vi "Factor multiply Parameter.vi"(9 "Factor to multiply":dbl[](array[numeric]), 10 "Z":i32[](array[numeric]), 11 "Param In":T1) -> (3 "Param Out":T1)   [LabVIEW 2023]
uses:
  control/Parameters.ctl
  c738a0e9-d9eb-444f-adff-f9f269ff3581.vi
  <vilib>/Comparison/Equal/Equal Functor/Equal Functor.lvclass
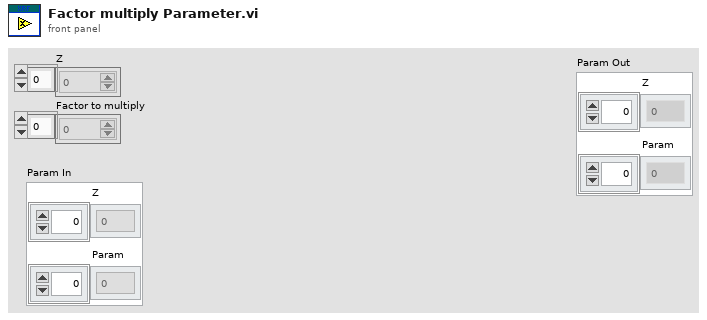
[diagram p1: front panel]
types:
  T1 = typedef "Parameters.ctl" = cluster{"Z":i32[], "Param":dbl[]}
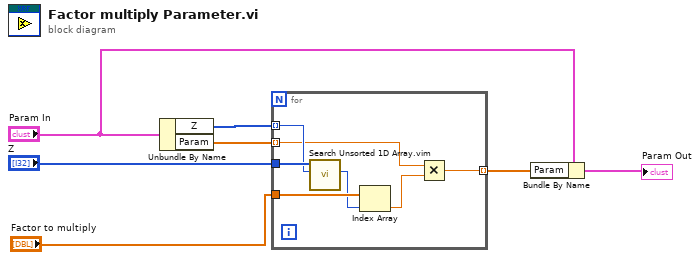
[diagram p0: block diagram]
diagram:
  n1 = Unbundle By Name("Param In") -> ("Z"=w5:i32[], "Param"=w4:dbl[])
  n2 = for {
    tunnel: "Z" -> [w13]
    tunnel: w5 -> [w12] mode=indexing
    tunnel: w4 -> [w9] mode=indexing
    tunnel: "Factor to multiply" -> [w14]
    tunnel: [w8] -> w6 mode=indexing
    n3 = call "Search Unsorted 1D Array.vim"("element"=w12, "unsorted 1D array"=w13) -> ("index of element"=w11:i32)  [unwired: 9 in]
    n4 = Index Array(array=w14, index=w11) -> (element=w10:dbl)
    n5 = Multiply(x=w9, y=w10) -> (x*y=w8:dbl)
  }
  n6 = Bundle By Name(cluster="Param In", "Param"=w6) -> (→"Param Out":T1)
